vi "Stop API handler.vi"(8 "error in (no error)":errorcluster) -> (0 "error out":errorcluster)   [LabVIEW 2020]
uses:
  <vilib>/addons/zeromq/socket_type.ctl
  global API.vi
  <vilib>/addons/zeromq/zeromq.lvlib
  <vilib>/addons/zeromq/zmq_context.lvclass
  <vilib>/addons/zeromq/zmq_socket.lvclass
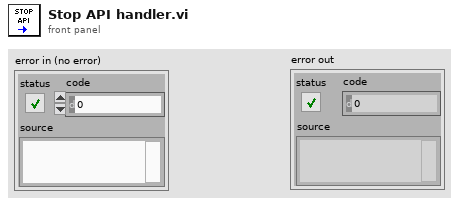
[diagram p1: front panel]
types:
  T1 = typedef "zeromq.lvlib/socket_type.ctl" = enum8{"ZMQ_PAIR", "ZMQ_PUB", "ZMQ_SUB", "ZMQ_REQ", "ZMQ_REP", "ZMQ_DEALER", "ZMQ_ROUTER", "ZMQ_PULL", "ZMQ_PUSH", "ZMQ_XPUB", "ZMQ_XSUB", "ZMQ_STREAM", "ZMQ_SERVER", "ZMQ_CLIENT", "ZMQ_RADIO", "ZMQ_DISH", "ZMQ_GATHER", "ZMQ_SCATTER", "ZMQ_DGRAM"}
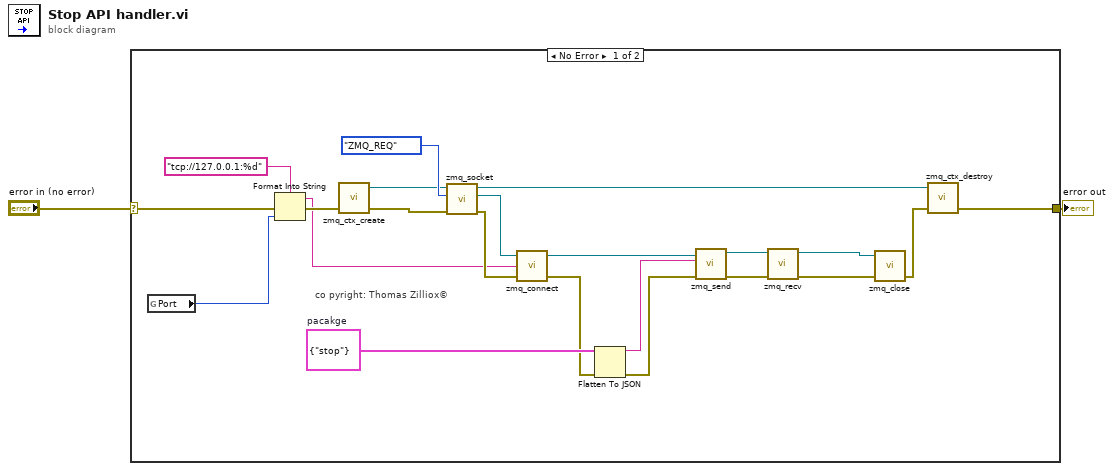
[diagram p0: block diagram]
diagram:
  n1 = case shown="No Error" "error in (no error)" {
    selector: "error in (no error)" -> [w16 w25]
    tunnel: [w13 w25] -> w1
    frame No Error {
      w8 = cluster{"message":string} {"message"="stop"}  # pacakge
      # "co pyright: Thomas Zilliox©"
      n2 = global read "global API.vi" "Port"() -> (w3:i32)
      n3 = Format Into String(format string="tcp://127.0.0.1:%d", error in=w16, w3) -> (resulting string=w4:string, error out=w14:errorcluster)  [unwired: 1 in]
      n4 = call <vilib>:"zmq_ctx_create.vi"("error in"=w14) -> ("error out"=w18:errorcluster, "context out"=w17:refnum<class "zmq_context.lvclass">)  [unwired: 3 in]
      n5 = call <vilib>:"zmq_socket.vi"("error in"=w18, "socket type"=socket_type."ZMQ_REQ", "context in"=w17) -> ("error out"=w22:errorcluster, "socket out"=w21:refnum<class "zmq_socket.lvclass">, "context out"=w20:refnum<class "zmq_context.lvclass">)  [unwired: 2 in]
      n6 = call <vilib>:"zmq_connect.vi"("error in"=w22, "endpoint"=w4, "socket in"=w21) -> ("error out"=w7:errorcluster, "socket out"=w23:refnum<class "zmq_socket.lvclass">)  [unwired: 1 in]
      n7 = Flatten To JSON(anything=w8, error in (no error)=w7) -> (JSON string=w5:string, 11:w6:errorcluster)  [unwired: 1 in]
      n8 = call <vilib>:"zmq_send.vi"("error in"=w6, "data"=w5, "socket in"=w23) -> ("error out"=w11:errorcluster, "socket out"=w12:refnum<class "zmq_socket.lvclass">)  [unwired: 4 in]
      n9 = call <vilib>:"zmq_recv.vi"("error in"=w11, "socket in"=w12) -> ("error out"=w10:errorcluster, "socket out"=w9:refnum<class "zmq_socket.lvclass">)  [unwired: 3 in, 3 out]
      n10 = call <vilib>:"zmq_close.vi"("error in"=w10, "socket"=w9) -> ("error out"=w24:errorcluster)  [unwired: 3 in]
      n11 = call <vilib>:"zmq_ctx_destroy.vi"("error in"=w24, "context in"=w20) -> ("error out"=w13:errorcluster)  [unwired: 3 in]
    }
    frame Error {
    }
  }
  "error out" <- w1
